vi "AlliGator Compute Basic Quantities.vi"(0 "Phasor Ratio (f1)":dbl, 1 "Data Information":T1, 5 "Reference Lifetime 1":dbl[unit], 7 "Reference Lifetime 2":dbl[unit], 9 "Complex Phasor":csg, 11 "error in (no error)":errorcluster, 12 "Phasor Frequency":dbl[unit], 13 "Compute Amplitude Ratio":bool) -> (4 "Average Lifetime":dbl, 8 "Basic Quantities":dbl[](array[numeric]), 15 "error out":errorcluster)   [LabVIEW 2021, in "AlliGator Phasor Ratio.lvlib"]
doc: "Computes phasor ratio-derived quantities."
uses:
  AlliGator Phasor Ratio.lvlib
  AlliGator Partial Data Information.ctl
  Phasor/Phasor.lvlib
  AlliGator Settings.lvlib
panel:
  # "see the AlliGator License on the block diagram (Ctrl+E or Window:Show Block Diagram)"
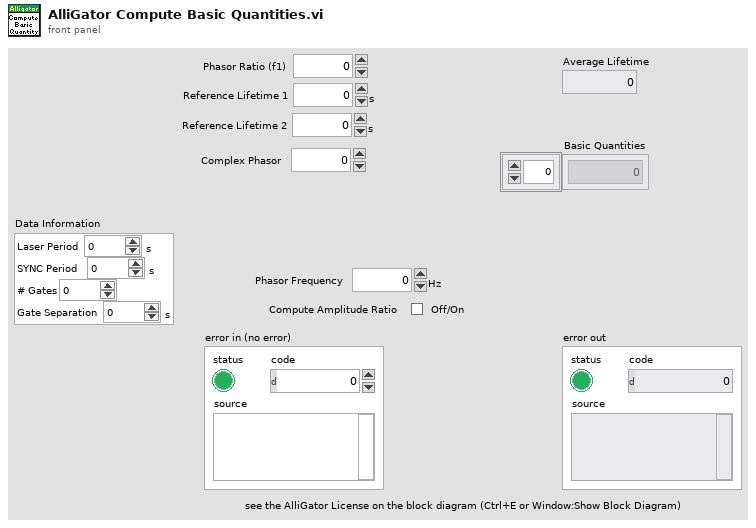
[diagram p1: front panel]
types:
  T1 = typedef "AlliGator Settings.lvlib/AlliGator Partial Data Information.ctl" = cluster{"Laser Period":dbl[unit], "SYNC Period":dbl[unit], "# Gates":u32, "Gate Separation":dbl[unit]}
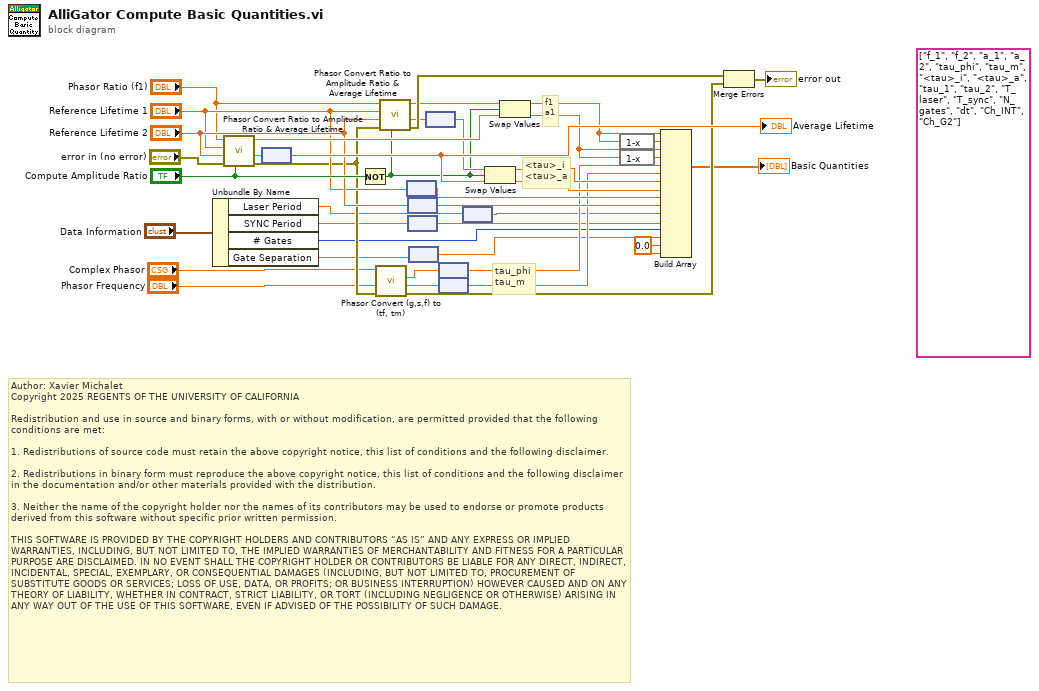
[diagram p0: block diagram]
diagram:
  w1 = 0.0 ("element")
  (unwired) string[] ["f_1", "f_2", "a_1", "a_2", "tau_phi", "tau_m", "<tau>_i", "<tau>_a", "tau_1", "tau_2", "T_laser", "T_sync", "N_gates", "dt", "Ch_INT", "Ch_G2"] ("Basic Variable Names")
  # "Author: Xavier Michalet\nCopyright 2025 REGENTS OF THE UNIVERSITY OF CALIFORNIA\n\nRedistribution and use in source and binary forms, with or without modification, are permitted provided that the following conditions are met:\n\n1. Redistributions of source code must retain the above copyright notice, this list of conditions and the following disclaimer.\n\n2. Redistributions in binary form must reproduce the above copyright notice, this list of conditions and the following disclaimer in the documentation and/or other materials provided with the distribution.\n\n3. Neither the name of the copyright holder nor the names of its contributors may be used to endorse or promote products derived from this software without specific prior written permission.\n\nTHIS SOFTWARE IS PROVIDED BY THE COPYRIGHT HOLDERS AND CONTRIBUTORS “AS IS” AND ANY EXPRESS OR IMPLIED WARRANTIES, INCLUDING, BUT NOT LIMITED TO, THE IMPLIED WARRANTIES OF MERCHANTABILITY AND FITNESS FOR A PARTICULAR PURPOSE ARE DISCLAIMED. IN NO EVENT SHALL THE COPYRIGHT HOLDER OR CONTRIBUTORS BE LIABLE FOR ANY DIRECT, INDIRECT, INCIDENTAL, SPECIAL, EXEMPLARY, OR CONSEQUENTIAL DAMAGES (INCLUDING, BUT NOT LIMITED TO, PROCUREMENT OF SUBSTITUTE GOODS OR SERVICES; LOSS OF USE, DATA, OR PROFITS; OR BUSINESS INTERRUPTION) HOWEVER CAUSED AND ON ANY THEORY OF LIABILITY, WHETHER IN CONTRACT, STRICT LIABILITY, OR TORT (INCLUDING NEGLIGENCE OR OTHERWISE) ARISING IN ANY WAY OUT OF THE USE OF THIS SOFTWARE, EVEN IF ADVISED OF THE POSSIBILITY OF SUCH DAMAGE."
  # "tau_phi\ntau_m"
  # "f1\na1"
  # "<tau>_i\n<tau>_a"
  n1 = Unbundle By Name("Data Information") -> ("Laser Period"=w8:dbl[unit], "SYNC Period"=w6:dbl[unit], "# Gates"=w4:u32, "Gate Separation"=w3:dbl[unit])
  n2 = call "Phasor Convert Ratio to Amplitude Ratio & Average Lifetime.vi"("Compute Amplitude Ratio"="Compute Amplitude Ratio", "error in (no error)"="error in (no error)", "Reference Lifetime 2"="Reference Lifetime 2", "Reference Lifetime 1"="Reference Lifetime 1", "Phasor Ratio (f1)"="Phasor Ratio (f1)") -> ("error out"=w34:errorcluster, "Average Lifetime"=w32:dbl[unit], "Phasor/Amplitude Ratio"=w38:dbl)  [unwired: 2 in, 2 out]
  n3 = node(w32) -> (w40:dbl)
  "Average Lifetime" <- w40
  n4 = Not(x="Compute Amplitude Ratio") -> (.not. x?=w15:bool)
  n5 = call "Phasor Convert (g,s,f) to (tf, tm).vi"("Error In"=w34, "Phasor Harmonic Frequency"="Phasor Frequency", "z"="Complex Phasor") -> ("Error Out"=w21:errorcluster, "Modulus Lifetime"=w24:dbl[unit], "Phase Lifetime"=w22:dbl[unit])  [unwired: 6 in]
  n6 = call "Phasor Convert Ratio to Amplitude Ratio & Average Lifetime.vi"("Compute Amplitude Ratio"=w15, "error in (no error)"=w34, "Reference Lifetime 2"="Reference Lifetime 2", "Reference Lifetime 1"="Reference Lifetime 1", "Phasor Ratio (f1)"="Phasor Ratio (f1)") -> ("error out"=w29:errorcluster, "Average Lifetime"=w14:dbl[unit], "Phasor/Amplitude Ratio"=w17:dbl)  [unwired: 2 in, 2 out]
  n7 = node("Reference Lifetime 1") -> (w30:dbl)
  n8 = node("Reference Lifetime 2") -> (w31:dbl)
  n9 = node(w6) -> (w5:dbl)
  n10 = node(w3) -> (w2:dbl)
  n11 = node(w14) -> (w16:dbl)
  n12 = node(w22) -> (w23:dbl)
  n13 = node(w24) -> (w25:dbl)
  n14 = node(w8) -> (w7:dbl)
  n15 = Swap Values(12:w16, 13:w15, 14:w40) -> (1:w27:dbl, 3:w28:dbl)
  n16 = Swap Values(12:w17, 13:w15, 14:w38) -> (1:w13:dbl, 3:w11:dbl)
  n17 = expression code="1-x"(w13) -> (w12:dbl)
  n18 = expression code="1-x"(w11) -> (w10:dbl)
  n19 = Build Array(w13, w12, w11, w10, w23, w25, w27, w28, w30, w31, w7, w5, w4, w2, w1, w1) -> (→"Basic Quantities":dbl[])
  n20 = Merge Errors(w29, w21) -> (→"error out":errorcluster)
